vi "Acquire.vi"(8 "error in":errorcluster, 9 "Timeout (ms)":i32, 10 "Digital capture samples":u32, 11 "gRPC session in":T1) -> (0 "error out":errorcluster, 2 "Digital waveform":u32[](array[numeric]), 3 "gRPC session out":T1)   [LabVIEW 2021, in "dcvmDPI_AD7606B_clientImpl.lvlib"]
uses:
  dcvmDPI_AD7606B_clientImpl.lvlib
  <vilib>/gRPC/LabVIEW gRPC Library/Shared/grpcId.ctl
  dcvmDPI_AD7606B_client/RPC Messages/dcvmDPI_AcquireRequest.ctl
  dcvmDPI_AD7606B_client/dcvmDPI_AD7606B_client.lvlib
  <vilib>/gRPC/LabVIEW gRPC Library/grpc-lvsupport-release.lvlib
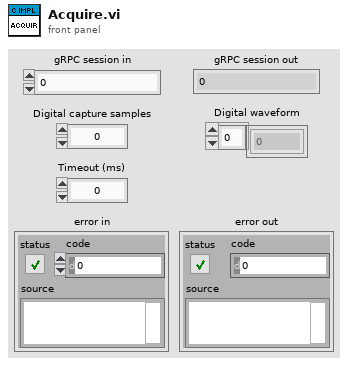
[diagram p1: front panel]
types:
  T1 = typedef "grpc-lvsupport-release.lvlib/grpcId.ctl" = u64
  T2 = typedef "dcvmDPI_AD7606B_client.lvlib/dcvmDPI_AcquireRequest.ctl" = cluster{"digital_capture_samples":u32, "timeout_ms":i32}
  T3 = typedef "dcvmDPI_AD7606B_client.lvlib/dcvmDPI_AcquireResponse.ctl" = cluster{"digital_waveform":u32[], "error":T4}
  T4 = typedef "dcvmDPI_AD7606B_client.lvlib/dcvmDPI_ErrorResponse.ctl" = cluster{"error_number":i32, "error_description":string}
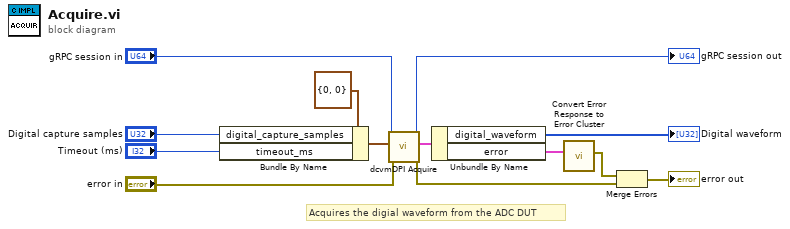
[diagram p0: block diagram]
diagram:
  # "Acquires the digial waveform from the ADC DUT"
  n1 = Bundle By Name(cluster=T2 {"digital_capture_samples"=0, "timeout_ms"=0} ("Request Data"), "digital_capture_samples"="Digital capture samples", "timeout_ms"="Timeout (ms)") -> (w10:T2)
  n2 = call "dcvmDPI Acquire.vi"("error in"="error in", "Request Data"=w10, "gRPC ID"="gRPC session in") -> ("error out"=w2:errorcluster, "Response Data"=w6:T3, "gRPC ID out"=→"gRPC session out":T1)  [unwired: 6 in]
  n3 = Unbundle By Name(w6) -> ("digital_waveform"=→"Digital waveform":u32[], "error"=w4:T4)
  n4 = call "Convert Error Response to Error Cluster.vi"("Error response"=w4) -> ("error out"=w3:errorcluster)  [unwired: 10 in]
  n5 = Merge Errors(w3, w2) -> (→"error out":errorcluster)
